vi "Compute Delta Best Fit Parameters from Hessian Matrix.vi"(4 "# Degrees of Freedom":i32, 6 "# Parameters":i32, 8 "Error In":errorcluster, 9 "CL Parameter":dbl, 10 "Chi2":dbl, 11 "Hessian":T1) -> (0 "Error Out":errorcluster, 3 "Delta Best Fit Parameters":dbl[](array[numeric]))   [LabVIEW 2021, in "Fits.lvlib"]
uses:
  Fits.lvlib
  <vilib>/Analysis/Matrix/Datatypes/RealMatrix.ctl
  <vilib>/gmath/statdist.llb/Student t Inverse CDF.vi
  <vilib>/Analysis/Matrix/Numeric/Conversions/Matrix To Array - RM.vi
  <vilib>/Analysis/Matrix/Numeric/Conversions/Array To Matrix - RA2.vi
  <vilib>/Analysis/baseanly.llb/Real Inverse Matrix.vi
  <vilib>/Analysis/NI_AALBase.lvlib
  <vilib>/gmath/NI_Gmath.lvlib
  Error/Error.lvlib
  <vilib>/Analysis/Matrix/NI_Matrix.lvlib
panel:
  # "see the AlliGator License on the block diagram (Ctrl+E or Window:Show Block Diagram)"
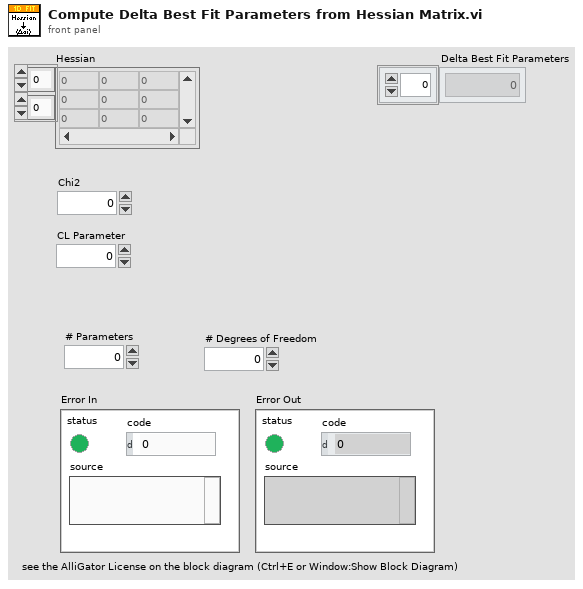
[diagram p1: front panel]
types:
  T1 = typedef "NI_Matrix.lvlib/RealMatrix.ctl" = dbl[][]
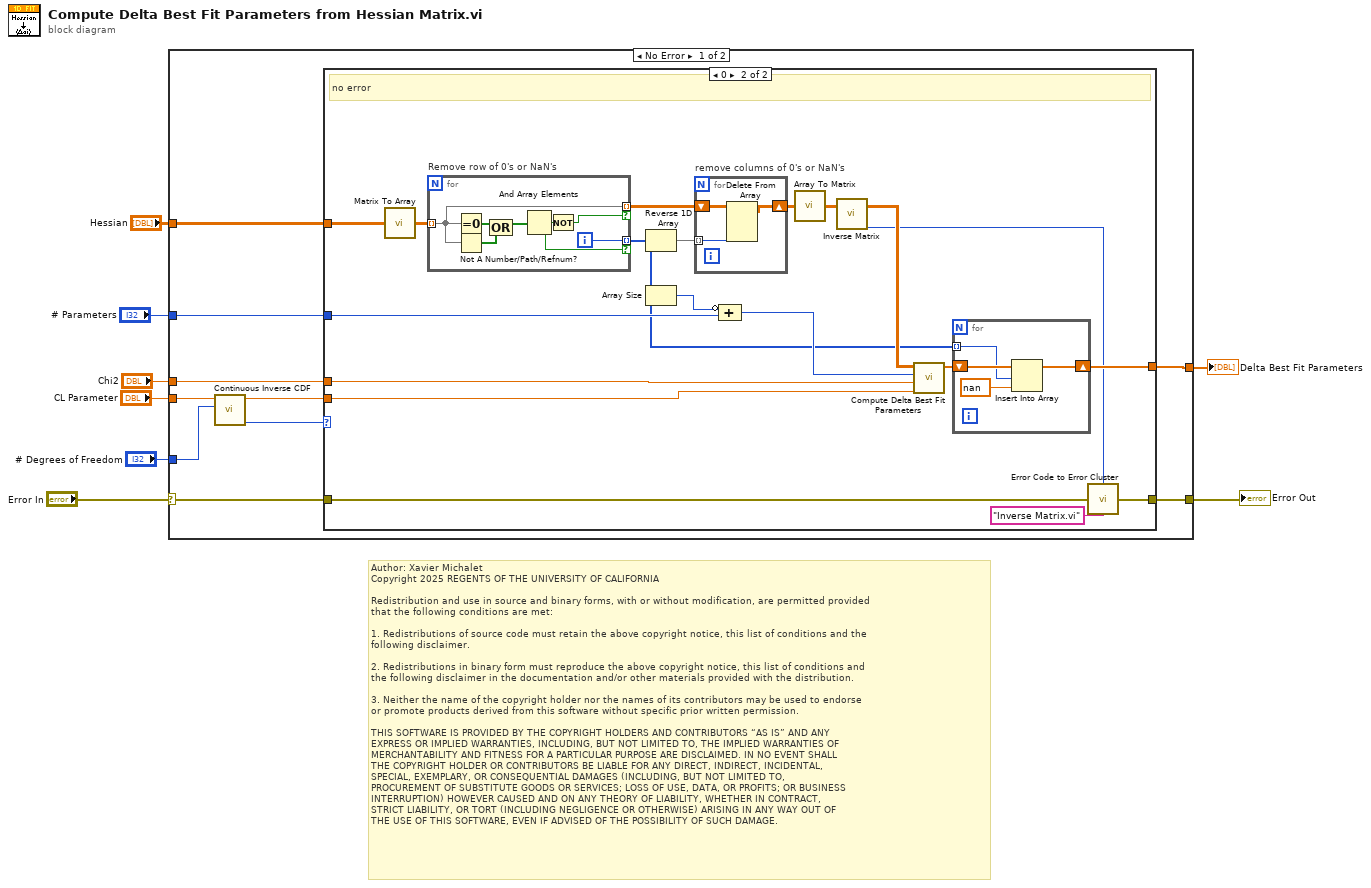
[diagram p0: block diagram]
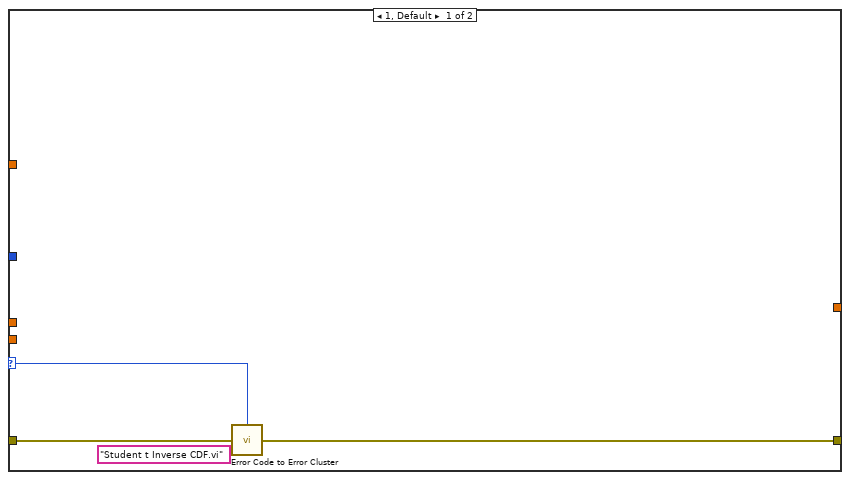
[diagram p2: hidden frame]
diagram:
  # "Author: Xavier Michalet\nCopyright 2025 REGENTS OF THE UNIVERSITY OF CALIFORNIA\n\nRedistribution and use in source and binary forms, with or without modification, are permitted provided\nthat the following conditions are met:\n\n1. Redistributions of source code must retain the above copyright notice, this list of conditions and the\nfollowing disclaimer.\n\n2. Redistributions in binary form must reproduce the above copyright notice, this list of conditions and\nthe following disclaimer in the documentation and/or other materials provided with the distribution.\n\n3. Neither the name of the copyright holder nor the names of its contributors may be used to endorse \nor promote products derived from this software without specific prior written permission.\n\nTHIS SOFTWARE IS PROVIDED BY THE COPYRIGHT HOLDERS AND CONTRIBUTORS “AS IS” AND ANY \nEXPRESS OR IMPLIED WARRANTIES, INCLUDING, BUT NOT LIMITED TO, THE IMPLIED WARRANTIES OF\nMERCHANTABILITY AND FITNESS FOR A PARTICULAR PURPOSE ARE DISCLAIMED. IN NO EVENT SHALL\nTHE COPYRIGHT HOLDER OR CONTRIBUTORS BE LIABLE FOR ANY DIRECT, INDIRECT, INCIDENTAL, \nSPECIAL, EXEMPLARY, OR CONSEQUENTIAL DAMAGES (INCLUDING, BUT NOT LIMITED TO, \nPROCUREMENT OF SUBSTITUTE GOODS OR SERVICES; LOSS OF USE, DATA, OR PROFITS; OR BUSINESS\nINTERRUPTION) HOWEVER CAUSED AND ON ANY THEORY OF LIABILITY, WHETHER IN CONTRACT, \nSTRICT LIABILITY, OR TORT (INCLUDING NEGLIGENCE OR OTHERWISE) ARISING IN ANY WAY OUT OF\nTHE USE OF THIS SOFTWARE, EVEN IF ADVISED OF THE POSSIBILITY OF SUCH DAMAGE."
  n1 = case shown="No Error" "Error In" {
    selector: "Error In" -> [w10 w56]
    tunnel: "# Parameters" -> [w18 _]
    tunnel: "Chi2" -> [w17 _]
    tunnel: [w16 _] -> w6
    tunnel: "Hessian" -> [w15 _]
    tunnel: "# Degrees of Freedom" -> [w14 _]
    tunnel: "CL Parameter" -> [w13 _]
    tunnel: [w9 w56] -> w1
    frame No Error {
      n2 = call-poly <vilib>:"Continuous Inverse CDF.vi"("k degrees of freedom"=w14, "cdf(x)"=w13) -> ("error"=w11:i32, "x"=w12:dbl)  [unwired: 8 in]
      n3 = case shown="0" w11 {
        selector: w11 -> [w21 _]
        tunnel: w18 -> [_ w41]
        tunnel: w17 -> [_ w40]
        tunnel: [_ w39] -> w16
        tunnel: w15 -> [_ w38]
        tunnel: w12 -> [_ w37]
        tunnel: w10 -> [w22 w36]
        tunnel: [w20 w35] -> w9
        frame 1, Default {
          n4 = call "Error Code to Error Cluster.vi"("Error Code"=w21, "Error Source"="Student t Inverse CDF.vi", "Error In"=w22) -> ("Error Out"=w20:errorcluster)  [unwired: 12 in]
        }
        frame 0 {
          # "no error"
          n5 = call-poly <vilib>:"Matrix To Array.vi"("Real Matrix"=w38) -> ("Real 2D Array"=w34:dbl[][])
          n6 = for "Remove row of 0's or NaN's" {
            tunnel: w34 -> [w51] mode=indexing
            tunnel: [w51] -> w33 mode=indexing if=w54
            tunnel: [w53] -> w26 mode=indexing if=w52
            i -> [w53]
            n7 = Equal To 0?(x=w51) -> (x = 0?=w55:bool[])
            n8 = Not A Number/Path/Refnum?(number/path/refnum=w51) -> (NaN/Path/Refnum?=w49:bool[])
            n9 = Compound Arithmetic op=OR(w55, w49) -> (w50:bool[])
            n10 = And Array Elements(Boolean array=w50) -> (logical AND=w52:bool)
            n11 = Not(x=w52) -> (.not. x?=w54:bool)
          }
          n12 = Reverse 1D Array(array=w26) -> (reversed array=w32:i32[])
          n13 = Array Size(array=w26) -> (size(s)=w28:i32)
          n14 = for "remove columns of 0's or NaN's" {
            tunnel: w32 -> [w46] mode=indexing
            shift-right: [w47] -> w31
            shift-left: w33 -> [w48]
            n15 = Delete From Array(array=w48, index (col)=w46) -> (array with subset deleted=w47:dbl[][])  [unwired: 2 in, 1 out]
          }
          n16 = Compound Arithmetic op=ADD(invert w28, w41) -> (w27:i32)
          n17 = call-poly <vilib>:"Array To Matrix.vi"("Real 2D Array"=w31) -> ("Real Matrix"=w30:T1)
          n18 = call-poly <vilib>:"Inverse Matrix.vi"("Input Matrix"=w30) -> ("error"=w24:i32, "Inverse Matrix"=w29:T1)  [unwired: 1 in]
          n19 = call "Compute Delta Best Fit Parameters.vi"("x"=w37, "Chi2"=w40, "# Parameters"=w27, "Covariance Matrix"=w29) -> ("Delta Best Fit Parameters"=w25:dbl[])  [unwired: 7 in]
          n20 = for {
            tunnel: w26 -> [w44] mode=indexing
            shift-right: [w42] -> w39
            shift-left: w25 -> [w45]
            n21 = Insert Into Array(array=w45, index=w44, new element=nan ("new element/subarray")) -> (w42:dbl[])
          }
          n22 = call "Error Code to Error Cluster.vi"("Error Code"=w24, "Error Source"="Inverse Matrix.vi", "Error In"=w36) -> ("Error Out"=w35:errorcluster)  [unwired: 12 in]
        }
      }
    }
    frame Error {
    }
  }
  "Delta Best Fit Parameters" <- w6
  "Error Out" <- w1
